vi "GetVIControlRef.vi"(8 "error in":errorcluster, 10 "Control Name":string="Current Starter Application", 11 "VI Ref In":refnum<vi>) -> (0 "error out":errorcluster, 2 "Control Reference":refnum<vi>, 3 "VI Ref Out":refnum<vi>)   [LabVIEW 2016]
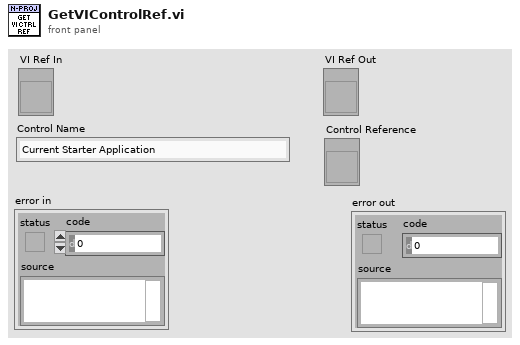
[diagram p1: front panel]
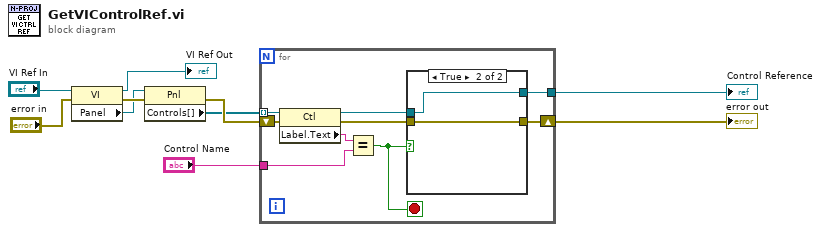
[diagram p0: block diagram]
diagram:
  n1 = property class="VI"(reference="VI Ref In", error in="error in") -> (reference out=→"VI Ref Out":refnum<vi>, error out=w9:errorcluster, "Panel"=w7:refnum<vi>)
  n2 = property class="Pnl"(reference=w7, error in=w9) -> (error out=w10:errorcluster, "Controls[]"=w8:refnum<vi>[])  [unwired: 1 out]
  n3 = for {
    tunnel: w8 -> [w19] mode=indexing
    tunnel: "Control Name" -> [w17]
    shift-right: [w13] -> w3
    shift-left: w10 -> [w15]
    tunnel: [w12] -> w1
    stop <- w11 stop-if-true
    n4 = property class="Ctl"(reference=w19, error in=w15) -> (reference out=w16:refnum<vi>, error out=w14:errorcluster, "Label.Text"=w18:string)
    n5 = Equal?(x=w18, y=w17) -> (x = y?=w11:bool)
    n6 = case shown="True" w11 {
      tunnel: w16 -> [_ w21]
      tunnel: [w20 w22] -> w13
      tunnel: w14 -> [w20 w22]
      tunnel: [_ w21] -> w12
      frame False {
      }
      frame True {
      }
    }
  }
  "Control Reference" <- w1
  "error out" <- w3
